vi "GetCleanSVNRevision.vi"(11 "File Path Control":path caption="File Path Control (leave blank to use Constants_Global value of EnFlo SW Folder)") -> (0 "isSVN":bool, 2 "svnDetails":string, 3 "svnRevision":string, 4 "Brief Output":string)   [LabVIEW 2022 SP3]
uses:
  Globals/Constants_global.vi
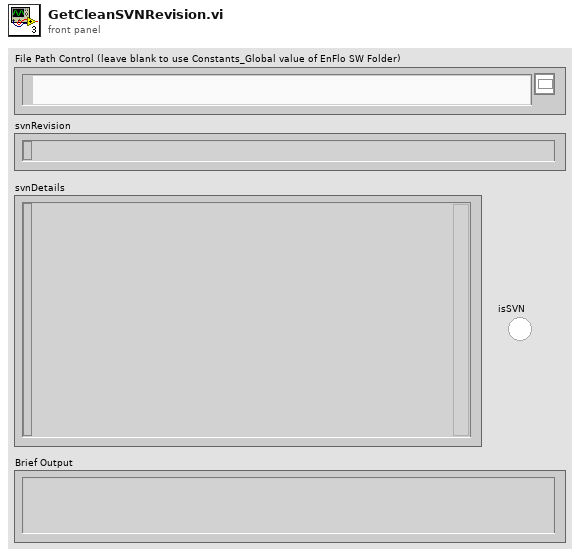
[diagram p1: front panel]
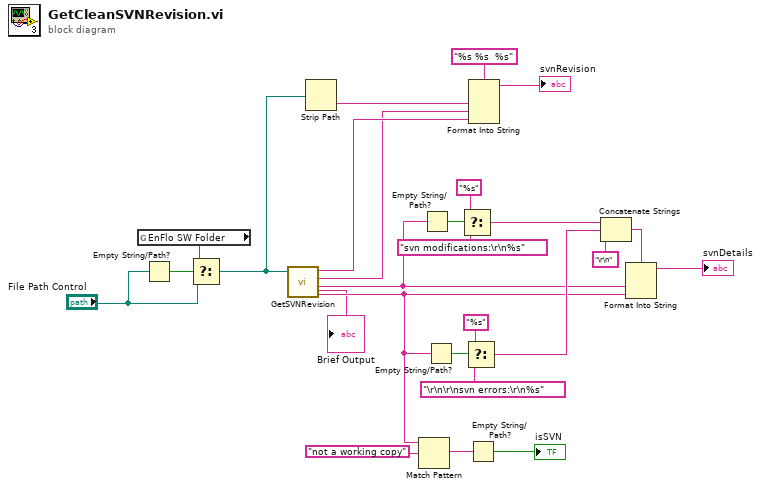
[diagram p0: block diagram]
diagram:
  n1 = global read "Constants_global.vi" "EnFlo SW Folder"() -> (w19:path)
  n2 = Empty String/Path?(string/path="File Path Control") -> (empty?=w20:bool)
  n3 = Select(t=w19, s=w20, f="File Path Control") -> (s? t:f=w17:path)
  n4 = call "GetSVNRevision.vi"("File Path Control"=w17) -> ("info&status error"=w5:string, "LocalModifications"=w6:string, "branch"=w3:string, "OverallRevision"=w4:string, "Brief Output"=→"Brief Output":string)  [unwired: 5 in, 1 out]
  n5 = Strip Path(path=w17) -> (name=w7:string)  [unwired: 1 out]
  n6 = Match Pattern(string=w5, regular expression="not a working copy") -> (match substring=w16:string)  [unwired: 1 in, 3 out]
  n7 = Empty String/Path?(string/path=w6) -> (empty?=w22:bool)
  n8 = Empty String/Path?(string/path=w5) -> (empty?=w25:bool)
  n9 = Select(t="%s", s=w22, f="svn modifications:\r\n%s" ("format string")) -> (s? t:f=w10:string)
  n10 = Select(t="%s" ("format string"), s=w25, f="\r\n\r\nsvn errors:\r\n%s" ("format string")) -> (s? t:f=w8:string)
  n11 = Empty String/Path?(string/path=w16) -> (empty?=→"isSVN":bool)
  n12 = Format Into String(format string="%s %s  %s" ("string"), w7, w3, w4) -> (resulting string=→"svnRevision":string)  [unwired: 2 in, 1 out]
  n13 = Concatenate Strings(w10, w8, "\r\n" ("string")) -> (w9:string)
  n14 = Format Into String(format string=w9, w6, w5) -> (resulting string=→"svnDetails":string)  [unwired: 2 in, 1 out]
